vi "NET Basic Serial Write and Read.vi"() -> ()   [LabVIEW 2009]
panel:
  in  "string to write":string="*IDN?\r\n"
  in  "write":bool=TRUE
  out "BytesRead":i32
  in  "read":bool=TRUE
  out "read string":string
  in  "Delay Before Read (ms)":u32=500
  in  "Handshaking":i32(ring)=2 items=["None", "XOnXOff", "RequestToSend", "RequestToSendXOnXOff"]
  in  "Stop Bits":i32(ring)=1 items=["None", "One", "Two", "OnePointFive"]
  in  "Data Bits":i32=8
  in  "Parity":i32(ring) items=["None", "Odd", "Even", "Mark", "Space"]
  in  "Baud Rate":i32=9600
  in  "Port Name":string="COM1"
  # "Select the serial resource and the operations (Read, Write, or both) to be performed.  If both are selected, the VI will write the data first, read data and then close the .NET reference that is opened to the port.  This VI will read any available data at the port."
  # "For additional information select File >> VI Properties >> Documentation"
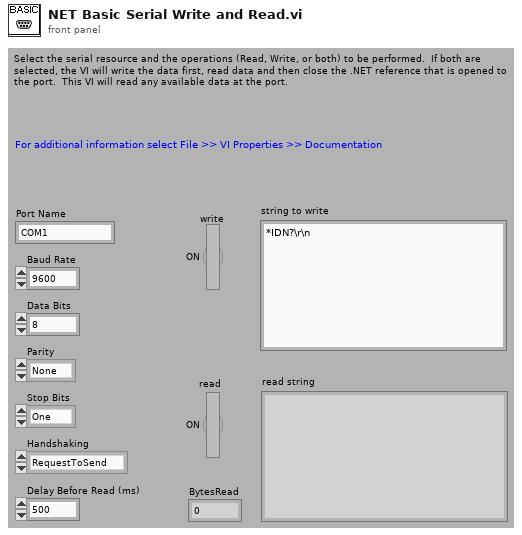
[diagram p1: front panel]
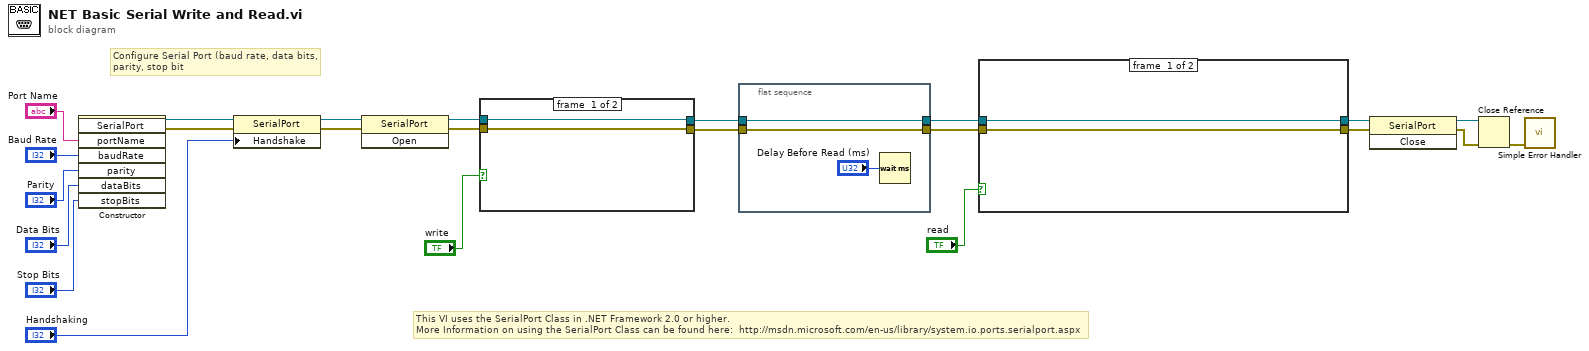
[diagram p0: block diagram]
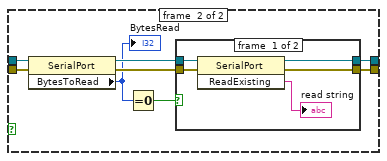
[diagram p2: hidden frame]
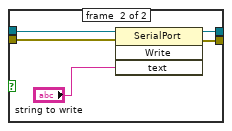
[diagram p4: hidden frame]
diagram:
  # "Configure Serial Port (baud rate, data bits,\nparity, stop bit"
  # "This VI uses the SerialPort Class in .NET Framework 2.0 or higher.\nMore Information on using the SerialPort Class can be found here:  http://msdn.microsoft.com/en-us/library/system.io.ports.serialport.aspx"
  n1 = constructor class="SerialPort"("portName"="Port Name", "baudRate"="Baud Rate", "parity"="Parity", "dataBits"="Data Bits", "stopBits"="Stop Bits") -> (reference out=w5:refnum<k24>, error out=w1:errorcluster)  [unwired: 3 in, 6 out]
  n2 = property class="SerialPort"(reference=w5, error in=w1, "Handshake"="Handshaking") -> (reference out=w4:refnum<k24>, error out=w3:errorcluster)
  n3 = invoke class="SerialPort" method="Open"(reference=w4, error in=w3) -> (reference out=w7:refnum<k24>, error out=w6:errorcluster)  [unwired: 1 in, 1 out]
  n4 = case shown="True" "write" {
    tunnel: [w25 w30] -> w18
    tunnel: [w24 w29] -> w17
    tunnel: w7 -> [w25 w27]
    tunnel: w6 -> [w24 w28]
    frame #0 {
    }
    frame #1 {
      n5 = invoke class="SerialPort" method="Write"(reference=w27, error in=w28, "text"="string to write") -> (reference out=w30:refnum<k24>, error out=w29:errorcluster)  [unwired: 1 in, 2 out]
    }
  }
  n6 = flat-sequence {
    tunnel: w18 -> [w33]
    tunnel: [w33] -> w16
    tunnel: [w32] -> w15
    tunnel: w17 -> [w32]
    frame #0 {
      n7 = Wait (ms)(milliseconds to wait="Delay Before Read (ms)") -> ()  [unwired: 1 out]
    }
  }
  n8 = case shown="True" "read" {
    tunnel: w16 -> [w35 w43]
    tunnel: w15 -> [w34 w42]
    tunnel: [w35 w39] -> w11
    tunnel: [w34 w38] -> w10
    frame #0 {
    }
    frame #1 {
      n9 = property class="SerialPort"(reference=w43, error in=w42) -> (reference out=w41:refnum<k24>, error out=w40:errorcluster, "BytesToRead"=w37:i32)
      "BytesRead" <- w37
      n10 = Equal To 0?(x=w37) -> (x = 0?=w36:bool)
      n11 = case shown="False" w36 {
        tunnel: w41 -> [w48 w50]
        tunnel: w40 -> [w47 w49]
        tunnel: [w46 w50] -> w39
        tunnel: [w45 w49] -> w38
        frame #0 {
          n12 = invoke class="SerialPort" method="ReadExisting"(reference=w48, error in=w47) -> (reference out=w46:refnum<k24>, error out=w45:errorcluster, "ReadExisting"=→"read string":string)  [unwired: 1 in]
        }
        frame #1 {
        }
      }
    }
  }
  n13 = invoke class="SerialPort" method="Close"(reference=w11, error in=w10) -> (reference out=w8:refnum<k24>, error out=w9:errorcluster)  [unwired: 1 in, 1 out]
  n14 = Close Reference(reference=w8, error in (no error)=w9) -> (error out=w14:errorcluster)
  n15 = call <vilib>:"Simple Error Handler.vi"("error in (no error)"=w14) -> ()  [unwired: 1 in, 8 out]
